vi "closeConnection.vi"(8 "error in (no error)":errorcluster, 11 "Arduino in":refnum<class "Arduino.lvclass">) -> (0 "error out":errorcluster, 3 "Arduino out":refnum<class "Arduino.lvclass">)   [LabVIEW 2020, in "Arduino.lvclass"]
uses:
  Arduino.lvclass
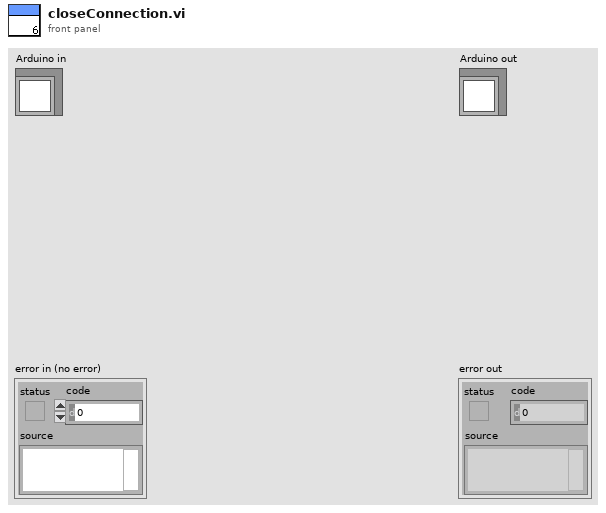
[diagram p1: front panel]
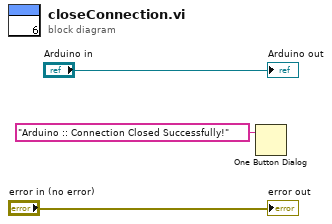
[diagram p0: block diagram]
diagram:
  n1 = One Button Dialog(message="Arduino :: Connection Closed Successfully!") -> ()  [unwired: 1 in, 1 out]
  "error out" <- "error in (no error)"
  "Arduino out" <- "Arduino in"
